vi "Run.vi"(8 "error in (no error)":errorcluster, 11 "Parameterized Test Suite In":refnum<class "Parameterized Test Suite.lvclass">) -> (0 "error out":errorcluster, 1 "Done?":bool, 2 "Results":T1(array[cluster]), 3 "Parameterized Test Suite Out":refnum<class "Parameterized Test Suite.lvclass">)   [LabVIEW 2020, in "Parameterized Test Suite.lvclass"]
doc: "Execute next test in suite. Done indicator is True if the test suite is exhausted and all active tests have been run."
uses:
  Parameterized Test Suite.lvclass
  Parameterized Test Suite.lvclass/Parameterized Test Suite.ctl
  <vilib>/Utility/miscctls.llb/LVMapReplaceAction.ctl
  <vilib>/Astemes/LUnit/Test Suite.lvclass
  C:/Program Files (x86)/National Instruments/LabVIEW 2020/vi.lib/Astemes/LUnit/Test Suite.lvclass
  C:/Program Files (x86)/National Instruments/LabVIEW 2020/vi.lib/Astemes/LUnit/LUnit Runnable.lvclass
  C:/git/astemes-lunit-parameterized-test/source/Parameterized Test Suite/Parameterized Test Suite.lvclass
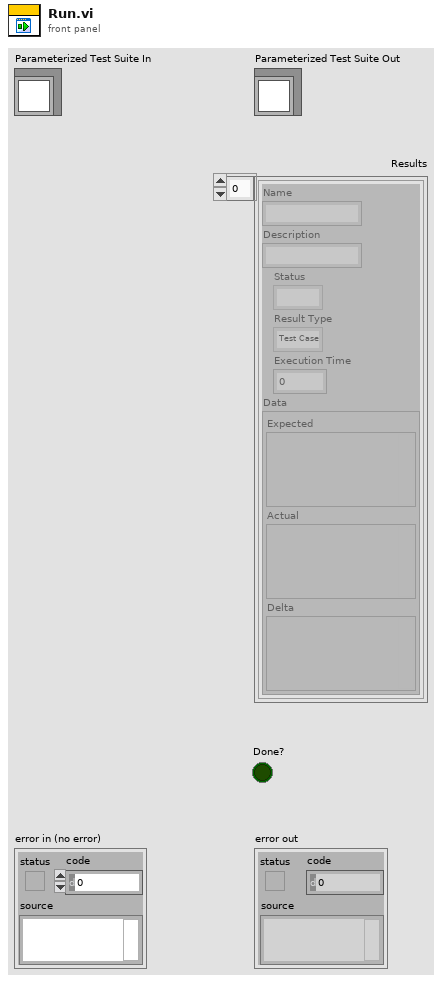
[diagram p1: front panel]
types:
  T1 = cluster{"Name":string, "Description":string, "Status":enum16{"", "Passed", "Failed", "Error", "Skipped", "Setup Error", "Broken", "Teardown Error"}, "Result Type":enum16{"Test Case", "Test Suite", "Test Run", "Pass", "Fail", "Skip", "Pass if", "Fail if", "Pass if Error", "Fail if Error", "Pass if Equal", "Fail if Equal"}, "Execution Time":dbl, "Data":cluster{"Expected":variant, "Actual":variant, "Delta":variant}}[]
  T2 = cluster{"Name":string, "Description":string, "Status":enum16{"", "Passed", "Failed", "Error", "Skipped", "Setup Error", "Broken", "Teardown Error"}, "Result Type":enum16{"Test Case", "Test Suite", "Test Run", "Pass", "Fail", "Skip", "Pass if", "Fail if", "Pass if Error", "Fail if Error", "Pass if Equal", "Fail if Equal"}, "Execution Time":dbl, "Data":cluster{"Expected":variant, "Actual":variant, "Delta":variant}}
  T3 = enum16{"Test Case", "Test Suite", "Test Run", "Pass", "Fail", "Skip", "Pass if", "Fail if", "Pass if Error", "Fail if Error", "Pass if Equal", "Fail if Equal"}
  T4 = enum16{"", "Passed", "Failed", "Error", "Skipped", "Setup Error", "Broken", "Teardown Error"}
  T5 = map{string, enum16{"", "Passed", "Failed", "Error", "Skipped", "Setup Error", "Broken", "Teardown Error"}}
  T6 = typedef "LVMapReplaceAction.ctl" = enum32{"Modify Entry only if found", "Add or Modify Entry", "Delete Entry"}
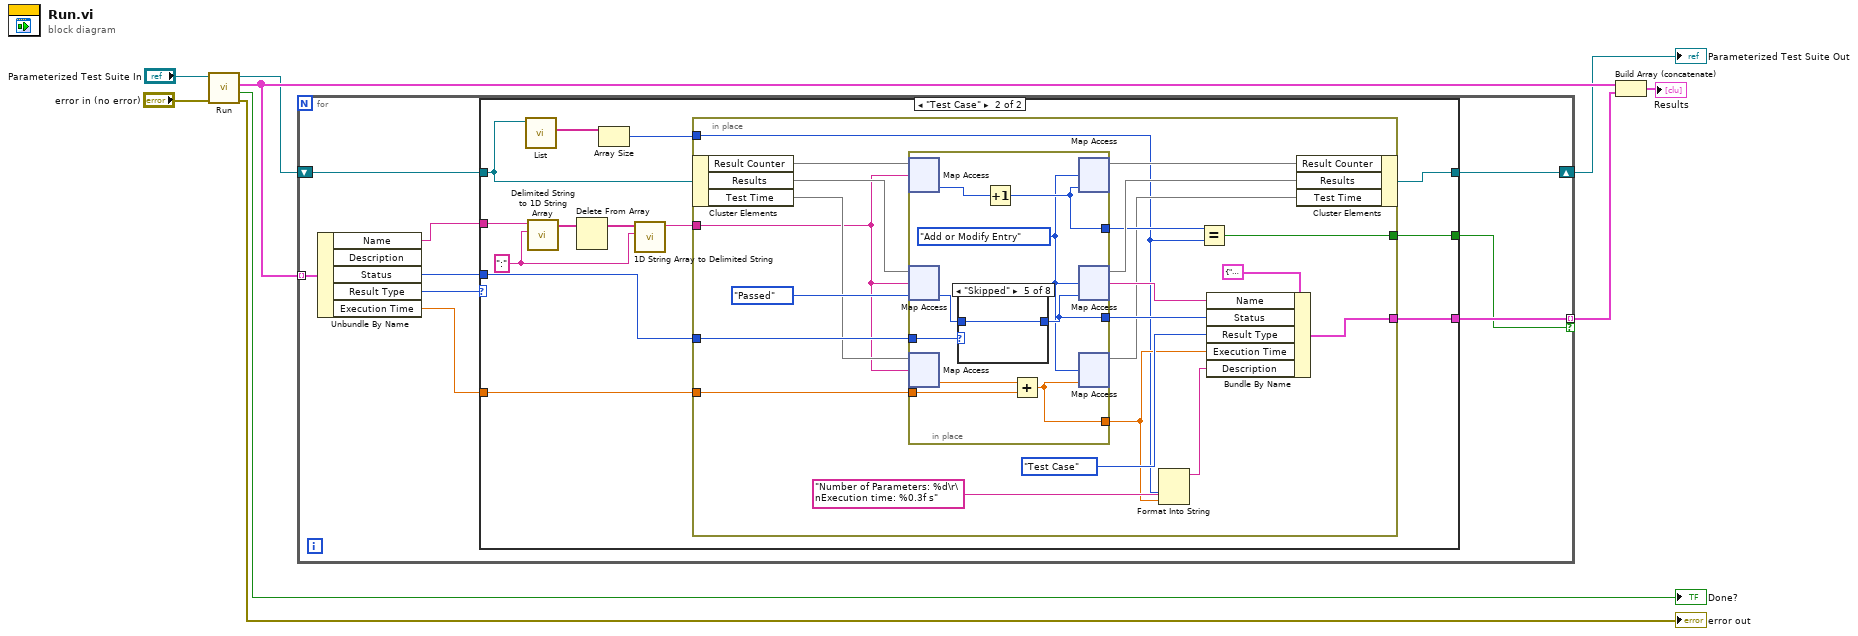
[diagram p0: block diagram]
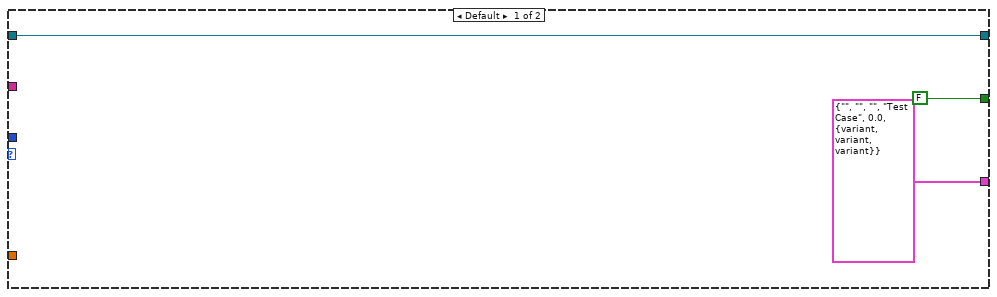
[diagram p2: hidden frame]
diagram:
  n1 = call-parent "Run.vi"("error in (no error)"="error in (no error)", "LUnit Test Suite In"="Parameterized Test Suite In") -> ("error out"=→"error out":errorcluster, "Done?"=→"Done?":bool, "Results"=w5:T1, "LUnit Test Suite In 2"=w4:refnum<class "Parameterized Test Suite.lvclass">)  [unwired: 6 in]
  n2 = for {
    tunnel: w5 -> [w18] mode=indexing
    shift-right: [w13] -> w3
    shift-left: w4 -> [w14]
    tunnel: [w12] -> w2 mode=indexing if=w11
    n3 = Unbundle By Name(w18) -> ("Name"=w16:string, "Status"=w15:T4, "Result Type"=w17:T3, "Execution Time"=w10:dbl)  [unwired: 1 out]
    n4 = case shown="\"Test Case\"" w17 {
      tunnel: w16 -> [_ w34]
      tunnel: w15 -> [_ w29]
      tunnel: w14 -> [w21 w23]
      tunnel: [w21 w28] -> w13
      tunnel: [T2 {"Name"="", "Description"="", "Status"=enum."", "Result Type"=enum."Test Case", "Execution Time"=0.0, "Data"={"Expected"=variant, "Actual"=variant, "Delta"=variant}} ("Results") w27] -> w12
      tunnel: [FALSE w26] -> w11
      tunnel: w10 -> [_ w25]
      frame Default {
      }
      frame "Test Case" {
        w31 = ":" ("delimiter")
        n5 = call <vilib>:"List.vi"("LUnit Test Suite In"=w23) -> ("List of Runnables"=w24:string[])  [unwired: 9 in, 1 out]
        n6 = call <vilib>:"Delimited String to 1D String Array.vi"("delimiter"=w31, "delimited string"=w34) -> ("string array"=w33:string[])  [unwired: 9 in]
        n7 = Delete From Array(array=w33) -> (array with subset deleted=w32:string[])  [unwired: 2 in, 1 out]
        n8 = Array Size(array=w24) -> (size(s)=w22:i32)
        n9 = call <vilib>:"1D String Array to Delimited String.vi"("delimiter"=w31, "string array"=w32) -> ("delimited string"=w30:string)  [unwired: 9 in]
        n10 = in-place {
          in-place-border: w30 -> [w40]
          in-place-border: w29 -> [w55]
          in-place-border: [w46] -> w27
          in-place-border: [w44] -> w26
          in-place-border: w25 -> [w41]
          in-place-border: w22 -> [w35]
          n11 = in-place-cluster #1(w23) -> ("Result Counter"=w53:map{string, i32}, "Results"=w52:T5, "Test Time"=w43:map{string, dbl})
          n12 = in-place {
            in-place-border: w55 -> [w63]
            in-place-border: [w61] -> w49
            in-place-border: [w60] -> w45
            in-place-border: w41 -> [w58]
            in-place-border: [w56] -> w38
            w59 = LVMapReplaceAction."Add or Modify Entry" ("action")
            n13 = in-place-map #2(w53, w40) -> (w64:i32)  [unwired: 1 in, 1 out]
            n14 = in-place-map #3(w52, w40, T4."Passed" ("Status")) -> (w62:T4)  [unwired: 1 out]
            n15 = in-place-map #4(w43, w40) -> (w57:dbl)  [unwired: 1 in, 1 out]
            n16 = case shown="\"Skipped\"" w63 {
              selector: w63 -> [_ _ w67 w68 _ w70 w71 w72]
              tunnel: w62 -> [w65 w66 _ _ w69 _ _ _]
              tunnel: [w65 w66 w67 w68 w69 w70 w71 w72] -> w61
              frame Default {
              }
              frame "Passed" {
              }
              frame "Failed" {
              }
              frame "Error" {
              }
              frame "Skipped" {
              }
              frame "Setup Error" {
              }
              frame "Broken" {
              }
              frame "Teardown Error" {
              }
            }
            n17 = Increment(x=w64) -> (x+1=w60:i32)
            n18 = Add(x=w57, y=w58) -> (x+y=w56:dbl)
            n19 = in-place-map #2(w60, w59) -> (w51:map{string, i32})  [unwired: 2 out]
            n20 = in-place-map #3(w61, w59) -> (w50:T5, w48:string)  [unwired: 1 out]
            n21 = in-place-map #4(w56, w59) -> (w42:map{string, dbl})  [unwired: 2 out]
          }
          n22 = Format Into String(format string="Number of Parameters: %d\r\nExecution time: %0.3f s", w35, w38) -> (resulting string=w37:string)  [unwired: 2 in, 1 out]
          n23 = Equal?(x=w45, y=w35) -> (x = y?=w44:bool)
          n24 = Bundle By Name(cluster=T2 {"Name"="", "Description"="", "Status"=enum."Passed", "Result Type"=enum."Test Case", "Execution Time"=0.0, "Data"={"Expected"=variant, "Actual"=variant, "Delta"=variant}} ("Results"), "Name"=w48, "Status"=w49, "Result Type"=T3."Test Case", "Execution Time"=w38, "Description"=w37) -> (w46:T2)
          n25 = in-place-cluster #1("Result Counter"=w51, "Results"=w50, "Test Time"=w42) -> (w28:refnum<class "Parameterized Test Suite.lvclass">)
        }
      }
    }
  }
  "Parameterized Test Suite Out" <- w3
  n26 = Build Array (concatenate)(w5, w2) -> (→"Results":T1)
